vi "Create measurement folder with date.vi"(7 "Operator":string, 8 "error in (no error)":errorcluster, 9 "system directory type":T1 items=["User Home"=0, "User Desktop"=1, "User Documents"=2, "User Application Data"=3, "User Preferences"=4, "User Temporary"=5, "Public Documents"=6, "Public Application Data"=7, "Public Preferences"=8, "Public Cache"=13, "System Core Libraries"=9, "System Installed Libraries"=10, "Application Files"=11, "Boot Volume Root"=12], 10 "Sample name":string, 11 "Subfolder":path) -> (0 "error out":errorcluster, 3 "dup path":path)   [LabVIEW 2017]
doc: "Create folder with current date, name of sampe and oprator in specified location.\nIf path is not specified, it creates measurement folder and subfolders with date, name of sample and operator. (users documents is default path)\nAll invalid characters will be replaced by dash.\nExample: C:\\Users\\JackieChan\\Documents\\Measurements\\2020\\2020-08-06 DPPH (Pikachu)\nIf operators name is empty, it will be ommited"
uses:
  <vilib>/Utility/sysdir.llb/System Directory Type.ctl
panel:
  out "Date":string
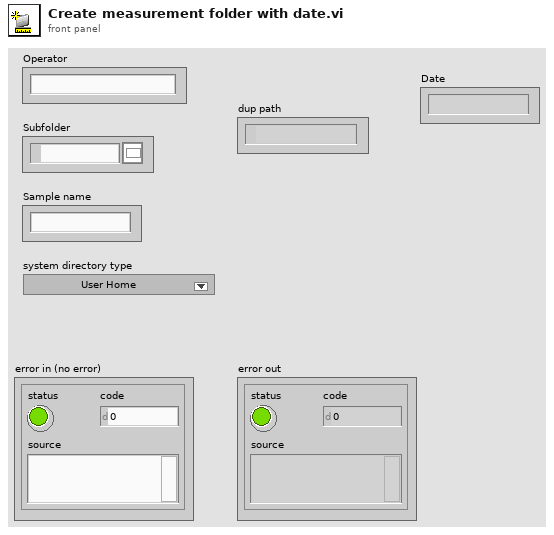
[diagram p1: front panel]
types:
  T1 = typedef "System Directory Type.ctl" = i32
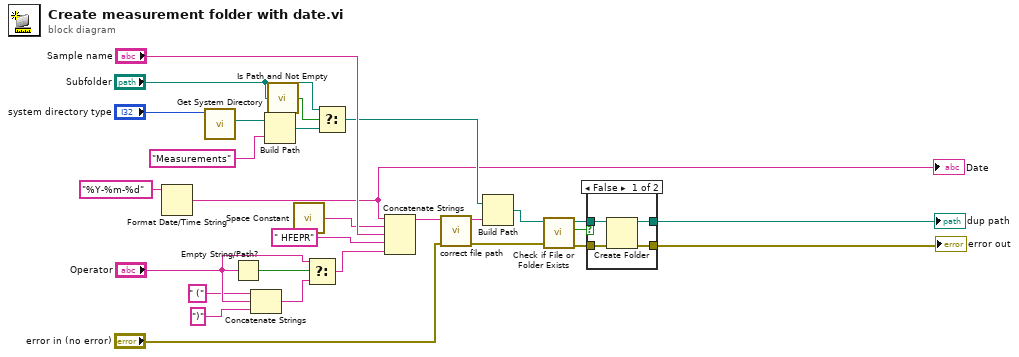
[diagram p0: block diagram]
diagram:
  n1 = Format Date/Time String(time format string (%c)="%Y-%m-%d") -> (date/time string=w3:string)  [unwired: 2 in]
  "Date" <- w3
  n2 = call <vilib>:"Get System Directory.vi"("system directory type"="system directory type") -> ("system directory"=w5:path)  [unwired: 10 in]
  n3 = Empty String/Path?(string/path="Operator") -> (empty?=w20:bool)
  n4 = Concatenate Strings(" (" ("string"), "Operator", ")" ("string")) -> (w23:string)
  n5 = Build Path(base path=w5, name or relative path="Measurements") -> (appended path=w12:path)
  n6 = call <vilib>:"Is Path and Not Empty.vi"("path"="Subfolder") -> ("Is Path and Not Empty?"=w9:bool)  [unwired: 4 in]
  n7 = call <vilib>:"Space Constant.vi"() -> ("String"=w18:string)
  n8 = Select(t="Operator", s=w20, f=w23) -> (s? t:f=w2:string)
  n9 = Select(t="Subfolder", s=w9, f=w12) -> (s? t:f=w11:path)
  n10 = Concatenate Strings(w3, w18, "Sample name", " HFEPR" ("string"), w2) -> (w25:string)
  n11 = call "correct file path.vi"("error in (no error)"="error in (no error)", "input path"=w25) -> ("error out"=w27:errorcluster, "corrected path"=w24:string)  [unwired: 8 in]
  n12 = Build Path(base path=w11, name or relative path=w24) -> (appended path=w16:path)
  n13 = call <vilib>:"Check if File or Folder Exists.vi"("error in (no error)"=w27, "path"=w16) -> ("error out"=w7:errorcluster, "file or folder exists?"=w6:bool, "dup path"=w8:path)  [unwired: 7 in]
  n14 = case shown="False" w6 {
    tunnel: w8 -> [w30 w34]
    tunnel: [w31 w33] -> w14
    tunnel: w7 -> [w32 w33]
    tunnel: [w29 w34] -> w13
    frame False {
      n15 = Create Folder(path (use dialog)=w30, error in=w32) -> (created path=w29:path, error out=w31:errorcluster)  [unwired: 1 in, 1 out]
    }
    frame True {
    }
  }
  "error out" <- w14
  "dup path" <- w13
